vi "YTO freq conversion_Naoj.vi"(0 "YTO desired frequency":sgl format="%.2f", 1 "YTO freq Min":sgl format="%.2f", 2 "YTO freq. Max":sgl format="%.2f") -> (18 "YTO Coarse tune":u16)   [LabVIEW 2017]
doc: "This VI converts a desired YTO frequency to YTO tune counts as specified in the ICD.\nInput parameters are;\n\nYTO freq. Min --- The maximum frequency of the YIG. Different range for each band and somewhat individual within a band.\n\nYTO freq. Max --- The maximum frequency of the YIG. Different range for each band and somewhat individual within a band.\n\nYTO desired frequency. --- The users desired frequency.\n\nOutput parameter is YTO tune count. This is a 12 bit vaue between 0 and 4095. The vaue is calculated using the formula;\n\nYTO Coarse tune = ((YTO_desired - YTO_f_min)/(YTO_f_max - YTO_f_min)) x 4095"
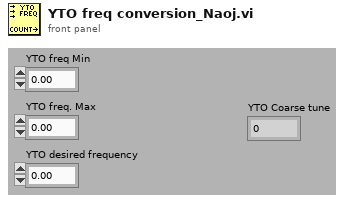
[diagram p1: front panel]
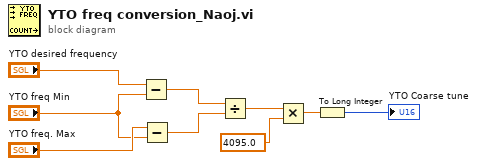
[diagram p0: block diagram]
diagram:
  n1 = Subtract(x="YTO desired frequency", y="YTO freq Min") -> (x-y=w6:sgl)
  n2 = Subtract(x="YTO freq. Max", y="YTO freq Min") -> (x-y=w5:sgl)
  n3 = Divide(x=w6, y=w5) -> (x/y=w4:sgl)
  n4 = Multiply(x=w4, y=4095.0) -> (x*y=w2:dbl)
  n5 = To Long Integer(number=w2) -> (32bit integer=→"YTO Coarse tune":i32)
